vi "passTestRobotKicksBall.vi"(6 "Thread organizer":T1, 11 "IA state":T3) -> (1 "Result":T1, 2 "Kicker robot":T2, 3 "Kicker robot":T2)   [LabVIEW 2017]
uses:
  <extravilib>/ChannelInstances/Lossy Stream-t'AI Input.ctl'/)Channel.ctl
  Core/AI Input.ctl
  Core/AI Robot.ctl
  Intel/Functions Enum.ctl
  Intel/AttackerStates.ctl
  Core/AI Ball.ctl
  Core/Field Size.ctl
  Core/AI Judge.ctl
  Intel/Command Enum.ctl
  Util/Events/Events.ctl
  <extravilib>/ChannelInstances/Lossy Stream-t'passTestStates.ctl'/)Channel.ctl
  passTestStates.ctl
  <extravilib>/ChannelInstances/Lossy Stream-dbl/)Channel.ctl
  <extravilib>/ChannelInstances/Lossy Stream-t'passTestStates.ctl'/Read With Abort.vi
  <extravilib>/ChannelInstances/Lossy Stream-t'AI Input.ctl'/Read With Abort.vi
  <extravilib>/ChannelInstances/Lossy Stream-dbl/Write With Abort.vi
  <extravilib>/ChannelInstances/Lossy Stream-t'passTestStates.ctl'/Write With Abort.vi
  <extravilib>/ChannelInstances/Lossy Stream-t'passTestStates.ctl'/EndpointRead.vi
  <extravilib>/ChannelInstances/Lossy Stream-t'AI Input.ctl'/EndpointRead.vi
  <extravilib>/ChannelInstances/Lossy Stream-dbl/Endpoint.vi
  <extravilib>/ChannelInstances/Lossy Stream-t'passTestStates.ctl'/Endpoint.vi
  <extravilib>/ChannelInstances/Lossy Stream-t'passTestStates.ctl'/)Channel.vi
  <resource>/ChannelSupport/_ChannelSupport/WaitIfNeeded.vi
  <extravilib>/ChannelInstances/Lossy Stream-t'AI Input.ctl'/)Channel.vi
  <extravilib>/ChannelInstances/Lossy Stream-dbl/)Channel.vi
  <extravilib>/ChannelInstances/Lossy Stream-t'passTestStates.ctl'.lvlib
  <extravilib>/ChannelInstances/Lossy Stream-t'AI Input.ctl'.lvlib
  <extravilib>/ChannelInstances/Lossy Stream-dbl.lvlib
panel:
  out "Kicker robot":dbl
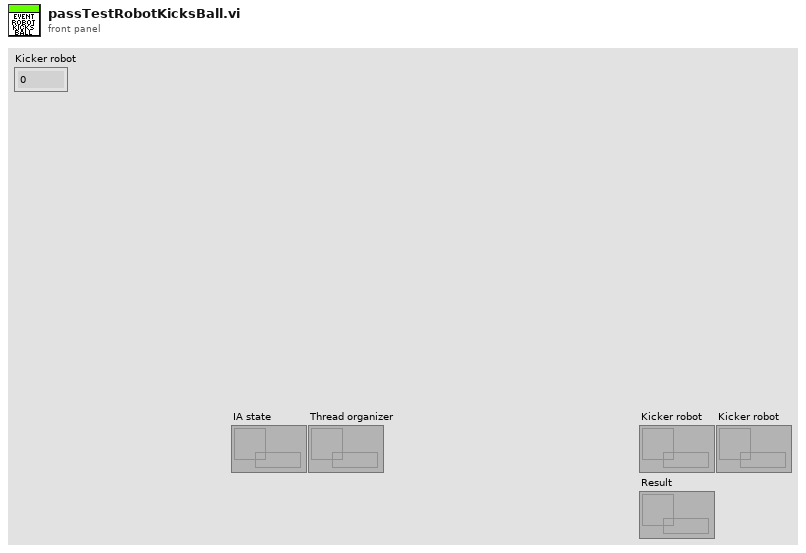
[diagram p1: front panel]
types:
  T1 = typedef "Lossy Stream-t'passTestStates.ctl'.lvlib/)Channel.ctl" = refnum<queue>
  T2 = typedef "Lossy Stream-dbl.lvlib/)Channel.ctl" = refnum<queue>
  T3 = typedef "Lossy Stream-t'AI Input.ctl'.lvlib/)Channel.ctl" = refnum<queue>
  T4 = typedef "passTestStates.ctl" = enum16{"Pass on the way", "Ball stops", "Pass intercepted", "Ball out of the field", "Ball missed robot", "Need more force to pass", "Too much force", "Correct pass", "Keep ball possesion", "Robot kicked the ball", "Waiting Kick", "Invalid: same robot", "Invalid: kicker ID 999", "Invalid: Receiver ID 999", "Invalid"}
  T5 = typedef "AI Input.ctl" = cluster{"our_robots":T6[], "enemy_robots":T6[], "balls":T9[], "geometry":T10, "IA Judge":T11, "Received Timestamp":timestamp, "Events":T13}
  T6 = typedef "AI Robot.ctl" = cluster{"id":u32, "function":T7, "x":dbl, "y":dbl, "orientation":dbl, "v_tangent":dbl, "v_normal":dbl, "v_ang":dbl, "kick_x":dbl, "kick_z":dbl, "dribble":bool, "Timestamp":timestamp, "dest_x":dbl, "dest_y":dbl, "dest_orientation":dbl, "estimatives":cluster{"est_v_tangent":dbl, "est_v_normal":dbl, "est_vx":dbl, "est_vy":dbl, "Pos Robot Est":dbl[]}, "dest_x_kick":dbl, "dest_y_kick":dbl, "Gap Coord":dbl[], "States":T8}
  T7 = typedef "Functions Enum.ctl" = enum16{"Attacker", "Goalie", "Defender", "Striker", "Goto 0", "Dummy", "Kicker", "ZigZag"}
  T8 = typedef "AttackerStates.ctl" = enum16{"Pass", "GoToTangent", "BallGetting", "GoToKick", ""}
  T9 = typedef "AI Ball.ctl" = cluster{"x":dbl, "y":dbl, "timestamp":timestamp, "Vel_x":dbl, "Vel_y":dbl, "Pos Bola Est":dbl[]}
  T10 = typedef "Field Size.ctl" = cluster{"line_width":u32, "field_length":u32, "field_width":u32, "boundary_width":u32, "referee_width":u32, "goal_width":u32, "goal_depth":u32, "goal_wall_width":u32, "center_circle_radius":u32, "defense_radius":u32, "defense_stretch":u32, "free_kick_from_defense_dist":u32, "penalty_spot_from_field_line_dist":u32, "penalty_line_from_spot_dist":u32}
  T11 = typedef "AI Judge.ctl" = cluster{"stage":string, "command":string, "our_goalie_id":dbl, "enemy_goalie_id":dbl, "command enum":T12, "Time":enum16{"Azul", "Amarelo"}}
  T12 = typedef "Command Enum.ctl" = enum16{"Halt", "Stop", "Force Start", "PKA Normal Start", "Prepare Kickoff Ally", "PKE Normal Start", "Prepare Kickoff Enemy", "Prepare Penalty Ally", "PPA Normal Start", "Prepare Penalty Enemy", "PPE Normal Start", "Direct Free Enemy", "Direct Free Ally", "Indirect Free Enemy", "Indirect Free Ally", "Timeout Enemy", "Timeout Ally", "Goal Enemy", "Goal Ally", "Ball Placement Enemy", "Ball Placement Ally", "Normal Half Time", "Extra Time Break", "Extra Half Time", "None", "Post Game"}
  T13 = typedef "Events.ctl" = cluster{"Touch":bool, "Ball out":bool, "id touch":dbl, "Ball out of \nVision":bool, "Ball inside \nGoalie area":bool, "Robot not responding":bool, "Robots responding status":dbl[], "Enemy Ball \nPossession":bool, "Pass State":bool, "id end of pass":dbl, "Kick":bool, "Id ini Possession":dbl, "Ball Possesion":bool, "Id Possesion":dbl}
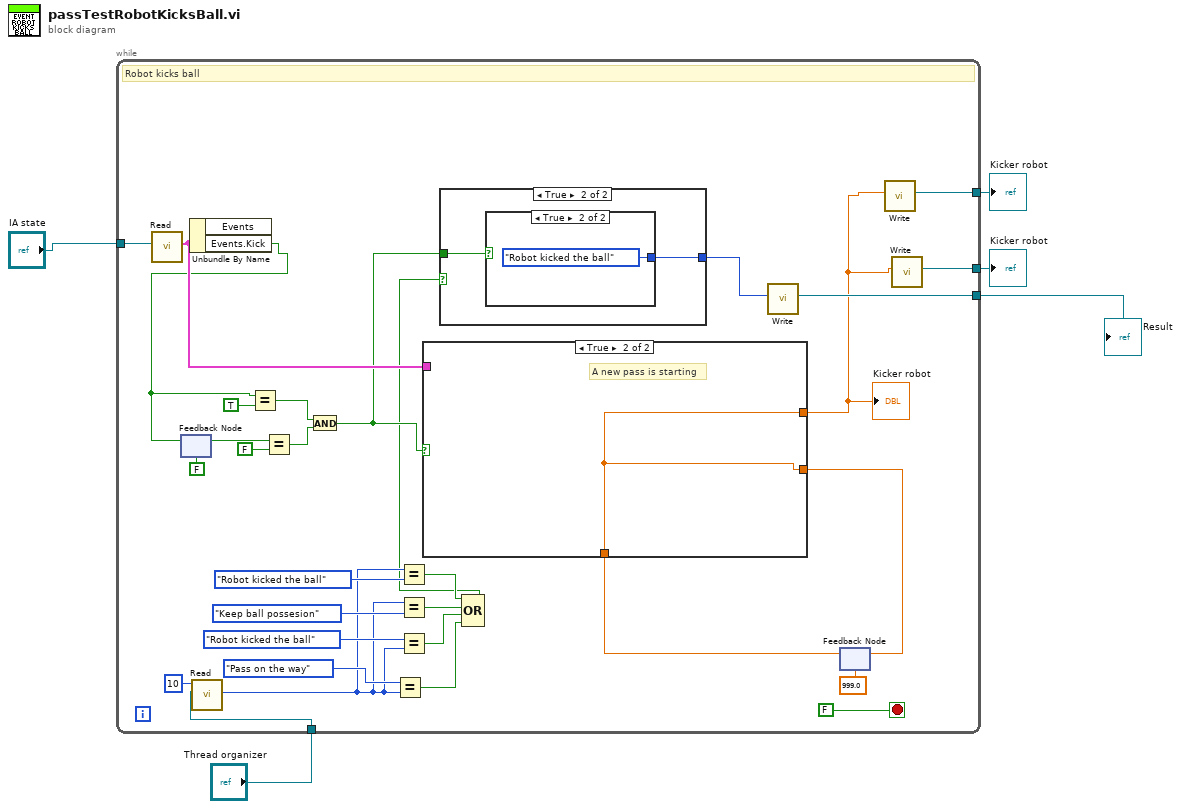
[diagram p0: block diagram]
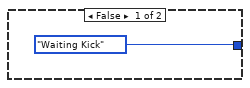
[diagram p2: hidden frame]
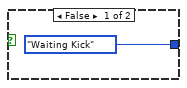
[diagram p3: hidden frame]
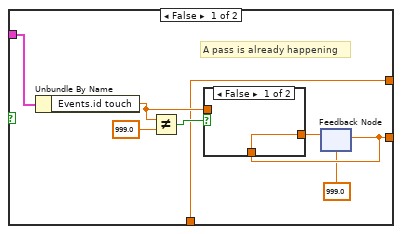
[diagram p4: hidden frame]
diagram:
  n1 = while {
    tunnel: [w35] -> w1
    tunnel: "IA state" -> [w33]
    tunnel: [w29] -> w3
    tunnel: "Thread organizer" -> [w20]
    tunnel: [w7] -> w2
    stop <- FALSE stop-if-true
    # "Robot kicks ball"
    n2 = call <extravilib>:"Read.vi"("channel"=w33) -> ("element"=w32:T5)  [unwired: 5 in, 5 out]
    n3 = feedback #1(FALSE ("Kick")) -> (w24:bool)
    n4 = Unbundle By Name(w32) -> ("Events.Kick"=w26:bool)  [unwired: 1 out]
    n5 = feedback-in #1(w26) -> ()
    n6 = call <extravilib>:"Read.vi"("channel"=w20, "timeout in ms (-1)"=10) -> ("element"=w10:T4)  [unwired: 4 in, 5 out]
    n7 = Equal?(x=w26, y=TRUE) -> (x = y?=w21:bool)
    n8 = Equal?(x=w24, y=FALSE) -> (x = y?=w22:bool)
    n9 = And(x=w21, y=w22) -> (x .and. y?=w19:bool)
    n10 = Equal?(x=passTestStates."Pass on the way" ("y"), y=w10) -> (x = y?=w14:bool)
    n11 = Equal?(x=w10, y=passTestStates."Robot kicked the ball") -> (x = y?=w11:bool)
    n12 = Equal?(x=w10, y=passTestStates."Keep ball possesion") -> (x = y?=w12:bool)
    n13 = Equal?(x=passTestStates."Robot kicked the ball" ("y"), y=w10) -> (x = y?=w13:bool)
    n14 = Compound Arithmetic op=OR(w11, w12, w13, w14) -> (w9:bool)
    n15 = case shown="True" w9 {
      tunnel: [passTestStates."Waiting Kick" w39] -> w34
      tunnel: w19 -> [_ w38]
      frame False {
      }
      frame True {
        n16 = case shown="True" w38 {
          tunnel: [passTestStates."Waiting Kick" passTestStates."Robot kicked the ball"] -> w39
          frame False {
          }
          frame True {
          }
        }
      }
    }
    n17 = call <extravilib>:"Write.vi"("element"=w34) -> ("channel"=w35:T1)  [unwired: 8 in, 2 out]
    n18 = feedback #2(999.0 ("id touch")) -> (w30:dbl)
    n19 = case shown="True" w19 {
      tunnel: w32 -> [w49 _]
      tunnel: [w44 w52] -> w31
      tunnel: w30 -> [w42 w52]
      tunnel: [w42 w52] -> w8
      frame False {
        # "A pass is already happening"
        n20 = Unbundle By Name(w49) -> ("Events.id touch"=w46:dbl)
        n21 = Not Equal?(x=w46, y=999.0) -> (x != y?=w47:bool)
        n22 = feedback #3(999.0 ("id touch")) -> (w44:dbl)
        n23 = case shown="False" w47 {
          tunnel: w46 -> [_ w51]
          tunnel: [w50 w51] -> w45
          tunnel: w44 -> [w50 _]
          frame False {
          }
          frame True {
          }
        }
        n24 = feedback-in #3(w45) -> ()
      }
      frame True {
        # "A new pass is starting"
      }
    }
    "Kicker robot" <- w8
    n25 = feedback-in #2(w31) -> ()
    n26 = call <extravilib>:"Write.vi"("element"=w8) -> ("channel"=w29:T2)  [unwired: 8 in, 2 out]
    n27 = call <extravilib>:"Write.vi"("element"=w8) -> ("channel"=w7:T2)  [unwired: 8 in, 2 out]
  }
  "Kicker robot" <- w3
  "Kicker robot" <- w2
  "Result" <- w1
